vi "Measure RPM 2.vi"(5 "Active":bool, 8 "error in":errorcluster, 11 "Knob in":refnum<vi>) -> (0 "error out":errorcluster, 1 "RPM Wfm":cluster{"X":dbl, "Y":dbl}[](array[cluster]), 2 "Raw":dbl[](array[numeric]) format="%0.2f", 3 "Median RPM":dbl format="%0.2f")   [LabVIEW 2017]
uses:
  <vilib>/DAQmx/read.llb/DAQmx Read (Counter 1D DBL 1Chan NSamp).vi
  <vilib>/DAQmx/miscellaneous.llb/DAQmx Fill In Error Info.vi
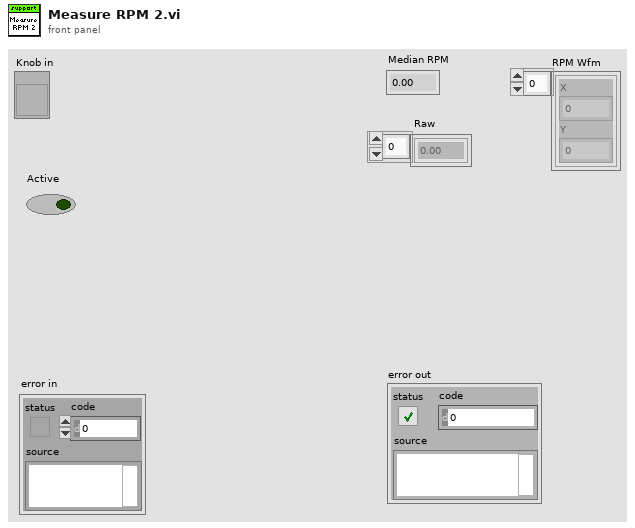
[diagram p1: front panel]
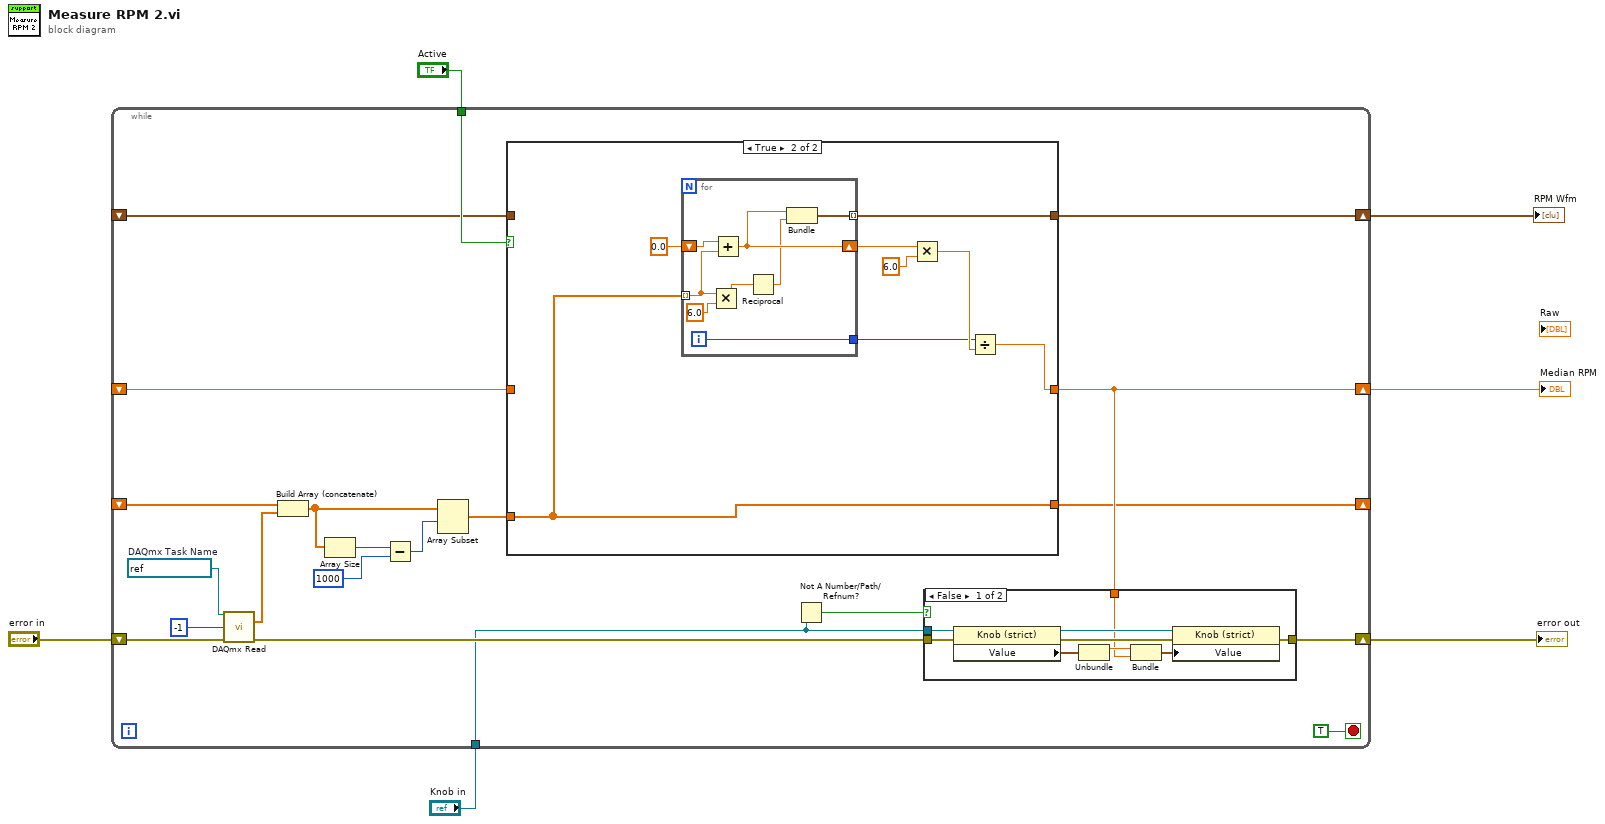
[diagram p0: block diagram]
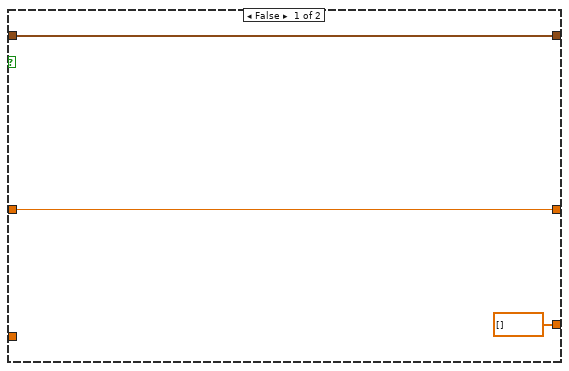
[diagram p3: hidden frame]
diagram:
  n1 = while {
    shift-right: [w13] -> w5
    shift-left: "error in" -> [w27]
    shift-right: [w8] -> _
    shift-left: _ -> [w24]
    tunnel: "Active" -> [w18]
    tunnel: "Knob in" -> [w15]
    shift-right: [w14] -> w3
    shift-left: _ -> [w11]
    shift-right: [w10] -> w1
    shift-left: _ -> [w9]
    stop <- TRUE stop-if-true
    w26 = refnum<k21> "PrecorCTR"  # DAQmx Task Name
    n2 = call-poly <vilib>:"DAQmx Read.vi"("task/channels in"=w26, "number of samples per channel"=-1, "error in"=w27) -> ("data"=w23:dbl[], "error out"=w16:errorcluster)  [unwired: 10 in, 1 out]
    n3 = Build Array (concatenate)(w24, w23) -> (w20:dbl[])
    n4 = Array Size(array=w20) -> (size(s)=w22:i32)
    n5 = Subtract(x=w22, y=1000) -> (x-y=w19:i32)
    n6 = Array Subset(array=w20, index=w19) -> (w7:dbl[])  [unwired: 1 in]
    n7 = case shown="True" w18 {
      tunnel: [w40 w42] -> w14
      tunnel: w11 -> [w40 _]
      tunnel: [w39 w47] -> w10
      tunnel: w9 -> [w39 _]
      tunnel: [dbl[] [] w46] -> w8
      tunnel: w7 -> [_ w46]
      frame False {
      }
      frame True {
        n8 = for {
          tunnel: w46 -> [w51] mode=indexing
          shift-right: [w55] -> w45
          shift-left: 0.0 -> [w56]
          tunnel: [w53] -> w47 mode=indexing
          tunnel: [w49] -> w41
          i -> [w49]
          n9 = Multiply(x=w51, y=6.0) -> (x*y=w52:dbl)
          n10 = Add(x=w56, y=w51) -> (x+y=w55:dbl)
          n11 = Reciprocal(x=w52) -> (1/x=w54:dbl)
          n12 = Bundle(w55, w54) -> (w53:cluster{dbl, dbl})  [unwired: 1 in]
        }
        n13 = Multiply(x=w45, y=6.0) -> (x*y=w43:dbl)
        n14 = Divide(x=w41, y=w43) -> (x/y=w42:dbl)
      }
    }
    n15 = Not A Number/Path/Refnum?(number/path/refnum=w15) -> (NaN/Path/Refnum?=w17:bool)
    n16 = case shown="False" w17 {
      tunnel: w16 -> [w35 w37]
      tunnel: [w30 w37] -> w13
      tunnel: w15 -> [w29 _]
      tunnel: w14 -> [w28 _]
      frame False {
        n17 = property class="Knob (strict)"(reference=w29, error in=w35) -> (reference out=w32:refnum<vi>, error out=w31:errorcluster, "Value"=w34:cluster{dbl, dbl})
        n18 = Unbundle(w34) -> (w36:dbl)  [unwired: 1 out]
        n19 = Bundle(w36, w28) -> (w33:cluster{dbl, dbl})  [unwired: 1 in]
        n20 = property class="Knob (strict)"(reference=w32, error in=w31, "Value"=w33) -> (error out=w30:errorcluster)  [unwired: 1 out]
      }
      frame True {
      }
    }
  }
  "error out" <- w5
  "Median RPM" <- w3
  "RPM Wfm" <- w1
